vi "LIDAR Test.vi"() -> ()   [LabVIEW 2016]
uses:
  <instrlib>/Hokuyo URG Series/Public/Initialize-Standard.vi
  <instrlib>/Hokuyo URG Series/Hokuyo URG Series.lvlib
panel:
  in  "polar attributes (hidden)":T1={"maximum"=30000.0, "minimum"=0.0, "clip to min"=FALSE, "log?(F)"=TRUE, "grid color"=6710886, "plot color"=65280, "fmt and prec"={"format"=enum."Decimal", "precision"=0}, "visible section"=8} {"minimum" format="%0.2f"; "maximum" format="%0.2f"}
  in  "Protocol":u32(ring)=2 items=["Convert to Latest", "SCIP 1.1", "SCIP 2.0"]
  in  "ID Query?":bool=TRUE
  in  "Checksum":bool
  in  "Stop":bool
  out "Data Aquired":picture
  in  "Grid Color":u32(colorbox)=16777222
  in  "Plot Color":u32(colorbox)=6618880
  in  "Max (m)":dbl=4.1
  in  "End Point":dbl=120.0
  in  "Start Point":dbl=-120.0
  in  "Cluster Count":dbl=1.0
  in  "Encoding Width":u16(ring)=3 items=["2 Byte"=2, "3 Byte"=3]
  in  "upper limit(-90-0)":dbl
  in  "upper limit(-90-0) 2":dbl
  out "Turn Right":bool
  out "Turn Left":bool
  out "Go straight/reverse":bool
  out "Left Wall points":i32
  out "Right wall points":i32
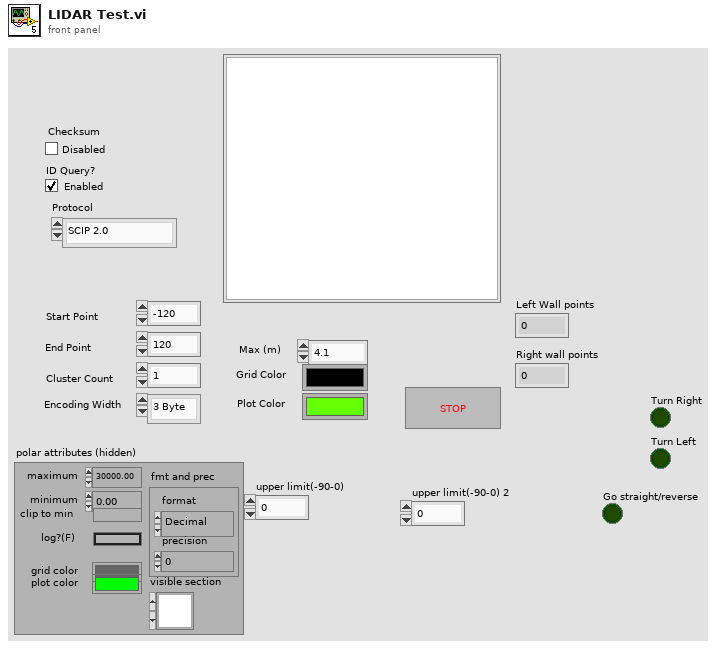
[diagram p1: front panel]
types:
  T1 = cluster{"maximum":dbl, "minimum":dbl, "clip to min":bool, "log?(F)":bool, "grid color":u32, "plot color":u32, "fmt and prec":cluster{"format":enum8{"Decimal", "Scientific", "Engineering", "Binary", "Octal", "Hex"}, "precision":u8}, "visible section":u16}
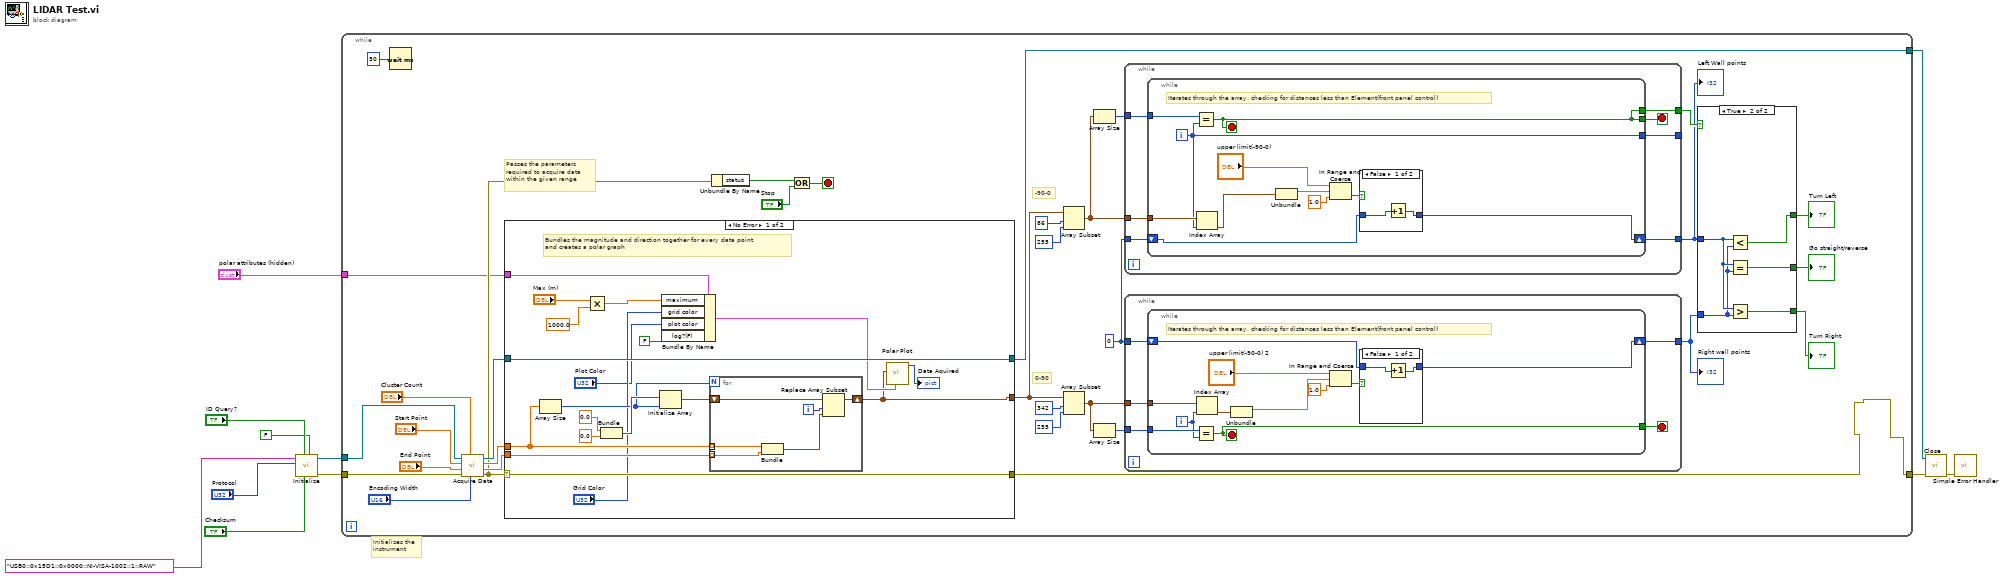
[diagram p0: block diagram]
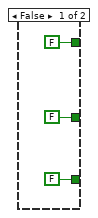
[diagram p2: hidden frame]
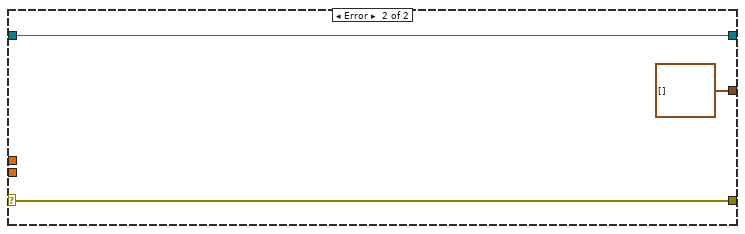
[diagram p5: hidden frame]
diagram:
  # "Initializes the instrument"
  n1 = call-poly <instrlib>:"Initialize.vi"("Reset? (F: No)"=FALSE ("Reset Instrument (Disabled)"), "Checksum (Disabled)"="Checksum", "ID Query? (Enabled)"="ID Query?", "Protocol (2: SCIP 2.0)"="Protocol", "VISA resource name"="USB0::0x15D1::0x0000::NI-VISA-1002::1::RAW") -> ("error out"=w3:errorcluster, "VISA resource name out"=w4:refnum<visa-resource-name>)  [unwired: 5 in]
  n2 = while {
    tunnel: w4 -> [w33]
    tunnel: [w12] -> w11
    tunnel: [w44] -> w5
    tunnel: w3 -> [w32]
    tunnel: "polar attributes (hidden)" -> [w31]
    stop <- w41 stop-if-true
    w17 = 0
    # "-90-0"
    # "0-90"
    # "Passes the parameters\nrequired to acquire data\nwithin the given range"
    n3 = Wait (ms)(milliseconds to wait=u32 50) -> ()  [unwired: 1 out]
    n4 = call <instrlib>:"Acquire Data.vi"("Data Encoding Width (3 Byte)"="Encoding Width", "Cluster Count (1)"="Cluster Count", "error in (no error)"=w32, "End Point (120°)"="End Point", "Start Point (-120°)"="Start Point", "VISA resource name"=w33) -> ("error out"=w37:errorcluster, "Direction"=w38:dbl[], "Magnitude"=w39:dbl[], "VISA resource name out"=w40:refnum<visa-resource-name>)  [unwired: 2 in]
    n5 = case shown="No Error" w37 {
      selector: w37 -> [w109 w120]
      tunnel: [w109 w120] -> w12
      tunnel: w40 -> [w110 w119]
      tunnel: [w110 w119] -> w44
      tunnel: w39 -> [w104 _]
      tunnel: w38 -> [w103 _]
      tunnel: w31 -> [w100 _]
      tunnel: [w93 cluster{dbl, dbl}[] []] -> w15
      frame No Error {
        # "Bundles the magnitude and direction together for every data point\nand creates a polar graph"
        n6 = Array Size(array=w104) -> (size(s)=w102:i32)
        n7 = Multiply(x="Max (m)", y=1000.0) -> (x*y=w96:dbl)
        n8 = Bundle(0.0, 0.0) -> (w106:cluster{dbl, dbl})  [unwired: 1 in]
        n9 = Initialize Array(w106, w102) -> (w105:cluster{dbl, dbl}[])
        n10 = Bundle By Name(cluster=w100, "maximum"=w96, "grid color"="Grid Color", "plot color"="Plot Color", "log?(F)"=FALSE) -> (w101:T1)
        n11 = for {
          N: w102 -> [_]
          shift-right: [w113] -> w93
          shift-left: w105 -> [w114]
          tunnel: w104 -> [w117] mode=indexing
          tunnel: w103 -> [w116] mode=indexing
          i -> [w115]
          n12 = Bundle(w117, w116) -> (w112:cluster{dbl, dbl})  [unwired: 1 in]
          n13 = Replace Array Subset(array=w114, new element=w112, index=w115) -> (w113:cluster{dbl, dbl}[])
        }
        n14 = call <vilib>:"Polar Plot.vi"("polar attributes"=w101, "data array [mag, phase (deg)]"=w93) -> ("new picture"=→"Data Aquired":picture)  [unwired: 9 in]
      }
      frame Error {
      }
    }
    n15 = Unbundle By Name(w37) -> ("status"=w43:bool)
    n16 = Or(x=w43, y="Stop") -> (x .or. y?=w41:bool)
    n17 = Array Subset(array=w15, index=86, length=255) -> (w24:cluster{dbl, dbl}[])
    n18 = Array Subset(array=w15, index=342, length=255) -> (w22:cluster{dbl, dbl}[])
    n19 = Array Size(array=w24) -> (size(s)=w23:i32)
    n20 = Array Size(array=w22) -> (size(s)=w21:i32)
    n21 = while {
      tunnel: w23 -> [w78]
      tunnel: w24 -> [w77]
      tunnel: [w75] -> _
      tunnel: [w74] -> w20
      tunnel: [w73] -> w18
      tunnel: w17 -> [w72]
      stop <- w76 stop-if-true
      n22 = while {
        tunnel: w78 -> [w89]
        tunnel: w77 -> [w88]
        tunnel: [w82] -> w76
        tunnel: [w83] -> w75
        tunnel: [w82] -> w74
        shift-right: [w81] -> w73
        shift-left: w72 -> [w84]
        i -> [w83]
        stop <- w82 stop-if-true
        # "Iterates through the array, checking for distances less than Element(front panel control)"
        n23 = Equal?(x=w89, y=w83) -> (x = y?=w82:bool)
        n24 = Index Array(array=w88, index=w83) -> (element=w87:cluster{dbl, dbl})
        n25 = Unbundle(w87) -> (w80:dbl)  [unwired: 1 out]
        n26 = In Range and Coerce(upper limit="upper limit(-90-0)", x=w80, lower limit=1.0) -> (In Range?=w85:bool)  [unwired: 1 out]
        n27 = case shown="False" w85 {
          tunnel: w84 -> [w91 w92]
          tunnel: [w90 w92] -> w81
          frame False {
            n28 = Increment(x=w91) -> (x+1=w90:i32)
          }
          frame True {
          }
        }
      }
    }
    "Left Wall points" <- w18
    n29 = while {
      tunnel: w21 -> [w57]
      tunnel: w22 -> [w56]
      tunnel: [w54] -> w19
      tunnel: w17 -> [w53]
      stop <- w55 stop-if-true
      n30 = while {
        tunnel: w57 -> [w68]
        tunnel: w56 -> [w67]
        tunnel: [w65] -> w55
        shift-right: [w60] -> w54
        shift-left: w53 -> [w61]
        i -> [w64]
        stop <- w65 stop-if-true
        # "Iterates through the array, checking for distances less than Element(front panel control)"
        n31 = Equal?(x=w68, y=w64) -> (x = y?=w65:bool)
        n32 = Index Array(array=w67, index=w64) -> (element=w66:cluster{dbl, dbl})
        n33 = Unbundle(w66) -> (w59:dbl)  [unwired: 1 out]
        n34 = In Range and Coerce(upper limit="upper limit(-90-0) 2", x=w59, lower limit=1.0) -> (In Range?=w62:bool)  [unwired: 1 out]
        n35 = case shown="False" w62 {
          tunnel: w61 -> [w70 w71]
          tunnel: [w69 w71] -> w60
          frame False {
            n36 = Increment(x=w70) -> (x+1=w69:i32)
          }
          frame True {
          }
        }
      }
    }
    "Right wall points" <- w19
    n37 = case shown="True" w20 {
      tunnel: w18 -> [_ w50]
      tunnel: w19 -> [_ w49]
      tunnel: [FALSE w52] -> w13
      tunnel: [FALSE w51] -> w16
      tunnel: [FALSE w48] -> w14
      frame False {
      }
      frame True {
        n38 = Less?(x=w50, y=w49) -> (x < y?=w48:bool)
        n39 = Equal?(x=w50, y=w49) -> (x = y?=w51:bool)
        n40 = Greater?(x=w50, y=w49) -> (0:w52:bool)
      }
    }
    "Turn Right" <- w13
    "Turn Left" <- w14
    "Go straight/reverse" <- w16
  }
  n41 = call <instrlib>:"Close.vi"("error in (no error)"=w11, "VISA resource name"=w5) -> ("error out"=w9:errorcluster)  [unwired: 9 in]
  n42 = call <vilib>:"Simple Error Handler.vi"("error in (no error)"=w9) -> ()  [unwired: 4 in, 5 out]
